vi "XML - Save to XML.vi"(8 "error in":errorcluster, 9 "Channel Groups":T1[](array[typedef]) {"Rx Channels"."Data Type" items=["U8", "U16", "U32", "U64", "I8", "I16", "I32", "I64", "SGL", "DBL", "EXT"]; "Tx Channels"."Data Type" items=["U8", "U16", "U32", "U64", "I8", "I16", "I32", "I64", "SGL", "DBL", "EXT"]}, 10 "XML Header Data":T3, 11 "XML File Path":path) -> (0 "error out":errorcluster)   [LabVIEW 2016, in "UDP-Custom-Device System Explorer.lvlib"]
uses:
  UDP-Custom-Device System Explorer.lvlib
  Types/XML/XML - Header Data.ctl
  Types/XML/XML - Group.ctl
  Types/XML/XML - Channel.ctl
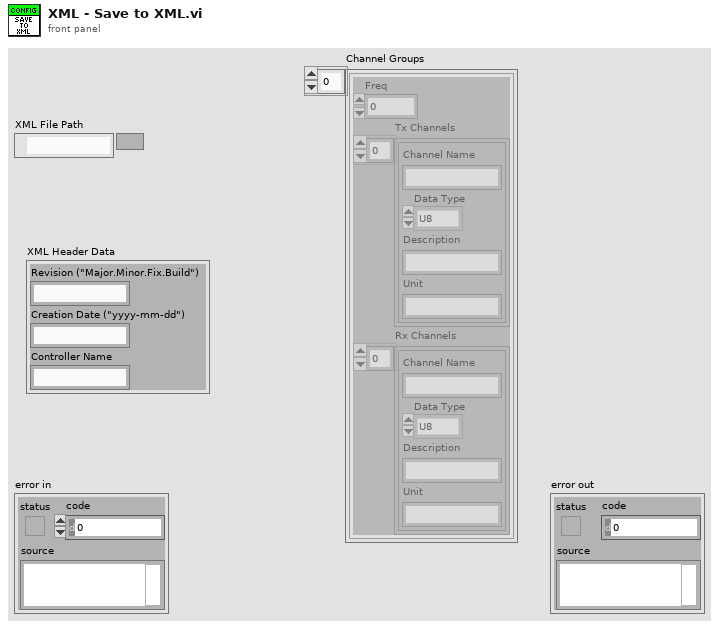
[diagram p1: front panel]
types:
  T1 = typedef "UDP-Custom-Device System Explorer.lvlib/XML - Group.ctl" = cluster{"Freq":i32, "Tx Channels":T2[], "Rx Channels":T2[]}
  T2 = typedef "UDP-Custom-Device System Explorer.lvlib/XML - Channel.ctl" = cluster{"Channel Name":string, "Data Type":u16, "Description":string, "Unit":string}
  T3 = typedef "UDP-Custom-Device System Explorer.lvlib/XML - Header Data.ctl" = cluster{"Revision (\"Major.Minor.Fix.Build\")":string, "Creation Date (\"yyyy-mm-dd\")":string, "Controller Name":string}
  T4 = enum16{"open", "replace", "create", "open or create", "replace or create", "replace or create with confirmation"}
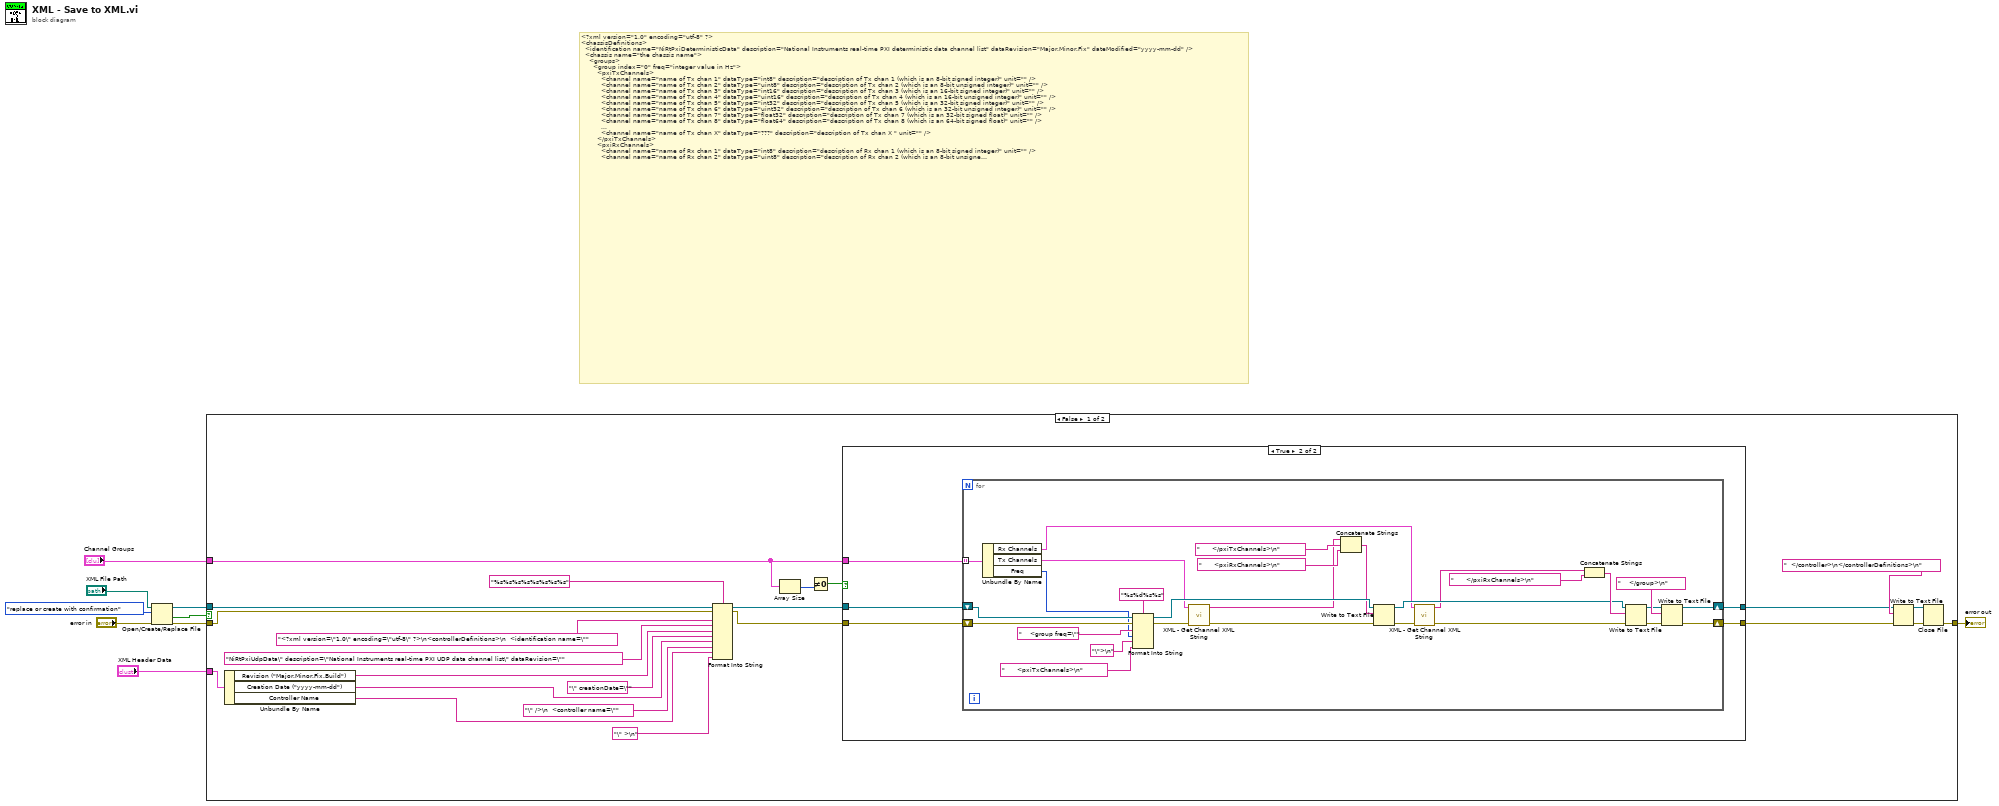
[diagram p0: block diagram]
diagram:
  # "<?xml version=\"1.0\" encoding=\"utf-8\" ?>\n<chassisDefinitions>\n  <identification name=\"NiRtPxiDeterministicData\" description=\"National Instruments real-time PXI deterministic data channel list\" dataRevision=\"Major.Minor.Fix\" dateModified=\"yyyy-mm-dd\" />\n  <chassis name=\"the chassis name\">\n    <groups>\n      <group index=\"0\" freq=\"integer value in Hz\">\n        <pxiTxChannels>\n          <channel name=\"name of Tx chan 1\" dataType=\"int8\" description=\"description of Tx chan 1 (which is an 8-bit signed integer)\" unit=\"\" />\n          <channel name=\"name of Tx chan 2\" dataType=\"uint8\" description=\"description of Tx chan 2 (which is an 8-bit unsigned integer)\" unit=\"\" />\n          <channel name=\"name of Tx chan 3\" dataType=\"int16\" description=\"description of Tx chan 3 (which is an 16-bit signed integer)\" unit=\"\" />\n          <channel name=\"name of Tx chan 4\" dataType=\"uint16\" description=\"description of Tx chan 4 (which is an 16-bit unsigned integer)\" unit=\"\" />\n          <channel name=\"name of Tx chan 5\" dataType=\"int32\" description=\"description of Tx chan 5 (which is an 32-bit signed integer)\" unit=\"\" />\n          <channel name=\"name of Tx chan 6\" dataType=\"uint32\" description=\"description of Tx chan 6 (which is an 32-bit unsigned integer)\" unit=\"\" />\n          <channel name=\"name of Tx chan 7\" dataType=\"float32\" description=\"description of Tx chan 7 (which is an 32-bit signed float)\" unit=\"\" />\n          <channel name=\"name of Tx chan 8\" dataType=\"float64\" description=\"description of Tx chan 8 (which is an 64-bit signed float)\" unit=\"\" />\n          ...\n          <channel name=\"name of Tx chan X\" dataType=\"???\" description=\"description of Tx chan X \" unit=\"\" />\n        </pxiTxChannels>\n        <pxiRxChannels>\n          <channel name=\"name of Rx chan 1\" dataType=\"int8\" description=\"description of Rx chan 1 (which is an 8-bit signed integer)\" unit=\"\" />\n          <channel name=\"name of Rx chan 2\" dataType=\"uint8\" description=\"description of Rx chan 2 (which is an 8-bit unsigned integer)\" unit=\"\" />\n          <channel name=\"name of Rx chan 3\" dataType=\"int16\" description=\"description of Rx chan 3 (which is an 16-bit signed integer)\" unit=\"\" />\n          <channel name=\"name of Rx chan 4\" dataType=\"uint16\" description=\"description of Rx chan 4 (which is an 16-bit unsigned integer)\" unit=\"\" />\n          <channel name=\"name of Rx chan 5\" dataType=\"int32\" description=\"description of Rx chan 5 (which is an 32-bit signed integer)\" unit=\"\" />\n          <channel name=\"name of Rx chan 6\" dataType=\"uint32\" description=\"description of Rx chan 6 (which is an 32-bit unsigned integer)\" unit=\"\" />\n          <channel name=\"name of Rx chan 7\" dataType=\"float32\" description=\"description of Rx chan 7 (which is an 32-bit signed float)\" unit=\"\" />\n          <channel name=\"name of Rx chan 8\" dataType=\"float64\" description=\"description of Rx chan 8 (which is an 64-bit signed float)\" unit=\"\" />\n          ...\n          <channel name=\"name of Rx chan X\" dataType=\"???\" description=\"description of Rx chan X\" unit=\"\" />\n        </pxiRxChannels>\n      </group>\n    </groups>\n  </chassis>\n</chassisDefinitions>"
  n1 = Open/Create/Replace File(file path (use dialog)="XML File Path", error in="error in", operation (0:open)=T4."replace or create with confirmation") -> (refnum out=w5:refnum<file>, cancelled=w7:bool, error out=w6:errorcluster)  [unwired: 3 in]
  n2 = case shown="False" w7 {
    tunnel: w6 -> [w30 w68]
    tunnel: w5 -> [w32 _]
    tunnel: "XML Header Data" -> [w27 _]
    tunnel: [w18 w68] -> w3
    tunnel: "Channel Groups" -> [w15 _]
    frame False {
      n3 = Unbundle By Name(w27) -> ("Revision (\"Major.Minor.Fix.Build\")"=w26:string, "Creation Date (\"yyyy-mm-dd\")"=w24:string, "Controller Name"=w22:string)
      n4 = Format Into String(format string="%s%s%s%s%s%s%s%s", initial string=w32, error in=w30, "<?xml version=\"1.0\" encoding=\"utf-8\" ?>\n<controllerDefinitions>\n  <identification name=\"", "NiRtPxiUdpData\" description=\"National Instruments real-time PXI UDP data channel list\" dataRevision=\"", w26, "\" creationDate=\"" ("input 4"), w24, "\" />\n  <controller name=\"", w22, "\" >\n") -> (resulting string=w13:refnum<file>, error out=w14:errorcluster)
      n5 = Array Size(array=w15) -> (size(s)=w17:i32)
      n6 = Not Equal To 0?(x=w17) -> (x != 0?=w16:bool)
      n7 = case shown="True" w16 {
        tunnel: w15 -> [_ w39]
        tunnel: w14 -> [w33 w37]
        tunnel: w13 -> [w34 w38]
        tunnel: [w33 w36] -> w12
        tunnel: [w34 w35] -> w11
        frame False {
        }
        frame True {
          n8 = for {
            tunnel: w39 -> [w67] mode=indexing
            shift-right: [w48] -> w35
            shift-left: w38 -> [w64]
            shift-right: [w49] -> w36
            shift-left: w37 -> [w65]
            n9 = Unbundle By Name(w67) -> ("Rx Channels"=w42:T2[], "Tx Channels"=w44:T2[], "Freq"=w62:i32)
            n10 = Format Into String(format string="%s%d%s%s", initial string=w64, error in=w65, "    <group freq=\"", w62, "\">\n", "      <pxiTxChannels>\n") -> (resulting string=w57:refnum<file>, error out=w47:errorcluster)
            n11 = call "XML - Get Channel XML String.vi"("error in (no error)"=w47, "Channels"=w44) -> ("error out"=w46:errorcluster, "Channels String"=w45:string)  [unwired: 8 in]
            n12 = Concatenate Strings(w45, "      </pxiTxChannels>\n", "      <pxiRxChannels>\n") -> (w56:string)
            n13 = Write to Text File(file (use dialog)=w57, text=w56, error in=w46) -> (refnum out=w50:refnum<file>, error out=w43:errorcluster)  [unwired: 1 in, 1 out]
            n14 = call "XML - Get Channel XML String.vi"("error in (no error)"=w43, "Channels"=w42) -> ("error out"=w40:errorcluster, "Channels String"=w41:string)  [unwired: 8 in]
            n15 = Concatenate Strings(w41, "      </pxiRxChannels>\n") -> (w54:string)
            n16 = Write to Text File(file (use dialog)=w50, text=w54, error in=w40) -> (refnum out=w52:refnum<file>, error out=w53:errorcluster)  [unwired: 1 in, 1 out]
            n17 = Write to Text File(file (use dialog)=w52, text="    </group>\n", error in=w53) -> (refnum out=w48:refnum<file>, error out=w49:errorcluster)  [unwired: 1 in, 1 out]
          }
        }
      }
      n18 = Write to Text File(file (use dialog)=w11, text="  </controller>\n</controllerDefinitions>\n", error in=w12) -> (refnum out=w19:refnum<file>, error out=w20:errorcluster)  [unwired: 1 in, 1 out]
      n19 = Close File(refnum=w19, error in=w20) -> (error out=w18:errorcluster)  [unwired: 1 out]
    }
    frame True {
    }
  }
  "error out" <- w3
